vi "Auto Controller.vi"(8 "Start Position":T2, 9 "End Position":T1, 10 "Cluster":cluster{"Start Time (ms)":u32, "Iterations":i32}, 11 "RobotDriveDevRef":T3) -> (1 "Finished?":bool, 2 "Right":dbl, 3 "Left":dbl)   [LabVIEW 2016]
uses:
  <vilib>/Rock Robotics/WPI/RobotDrive/WPI_RobotDriveDevRef.ctl
  <vilib>/Rock Robotics/WPI/MotorControl/WPI_MotorControlDeviceRef.ctl
  <vilib>/Rock Robotics/WPI/MotorControl/WPI_MotorControlType.ctl
  <vilib>/Rock Robotics/SystemInterfaces/DIO/FPGA_DIOPWMChannel.ctl
  <vilib>/Rock Robotics/WPI/PWM/WPI_PWMDeadband.ctl
  Shared/AutoPositions Type Def.ctl
  Shared/AutoEndPosition Type Def.ctl
  <vilib>/Rock Robotics/WPI/Camera/WPI_CameraExposure Values.ctl
  NavX/NavX Global.vi
  <vilib>/Rock Robotics/Network Tables/NT Read Number.vi
  Framework/Robot Global Data.vi
  <vilib>/Rock Robotics/Network Tables/NT Write Number.vi
panel:
  out "Straight 3":u32
  out "Turn 3":u32
  out "Drive To Center":u32
  out "Turn 2":u32
  out "Backup 1":u32
  out "Release Gear":u32
  out "Straight 2":u32
  out "Turn 1 Correction":u32
  out "Turn 1":u32
  out "Straight 1":u32
  # "Side Gear Auto"
  # "Center Auto"
  # "Shoot Auto"
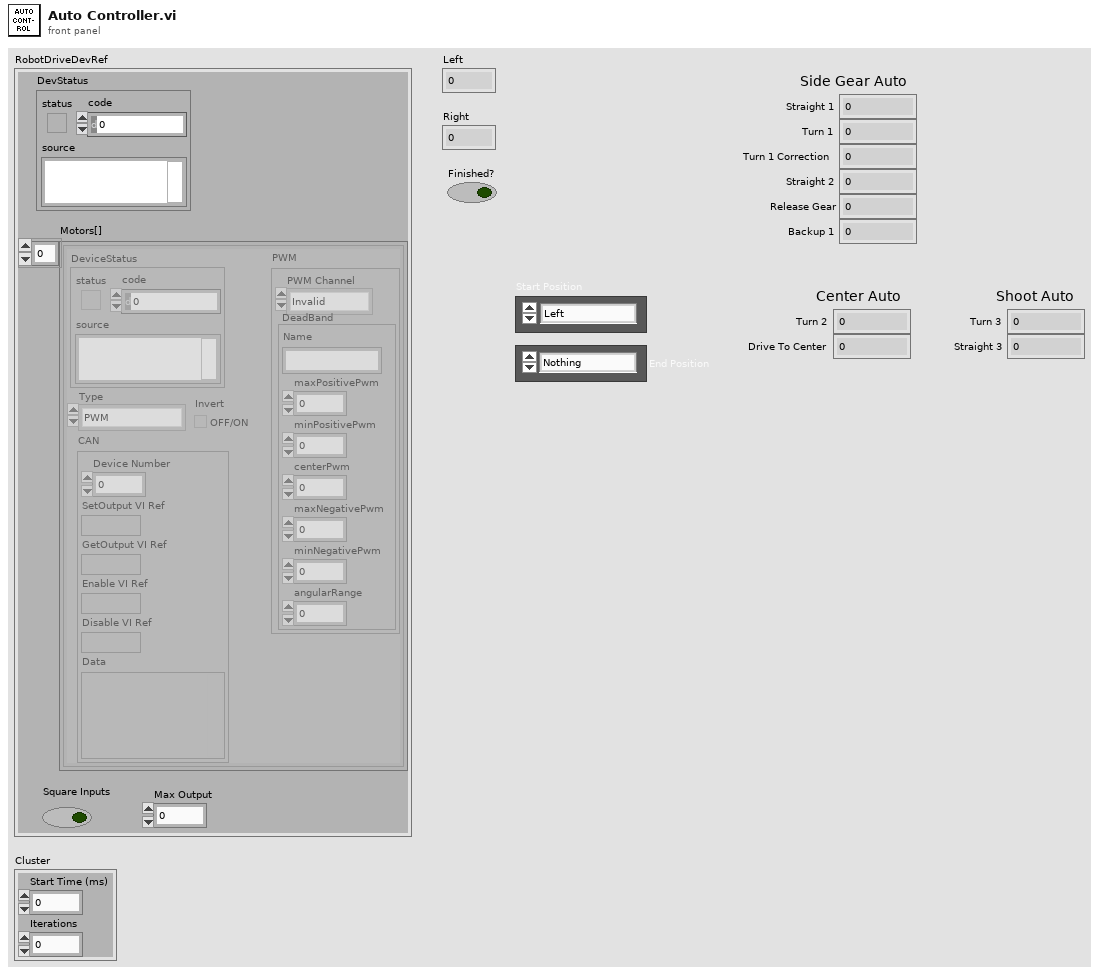
[diagram p1: front panel]
types:
  T1 = typedef "AutoEndPosition Type Def.ctl" = enum16{"Nothing", "Center", "Shoot"}
  T2 = typedef "AutoPositions Type Def.ctl" = enum16{"Left", "Middle", "Right"}
  T3 = typedef "WPI_RobotDriveDevRef.ctl" = cluster{"DevStatus":errorcluster, "Motors[]":T4[], "Square Inputs":bool, "Max Output":dbl}
  T4 = typedef "WPI_MotorControlDeviceRef.ctl" = cluster{"DeviceStatus":errorcluster, "Type":T5, "PWM":cluster{"PWM Channel":T6, "DeadBand":T7}, "CAN":cluster{"Device Number":u8, "SetOutput VI Ref":variant, "GetOutput VI Ref":variant, "Enable VI Ref":variant, "Disable VI Ref":variant, "Data":variant}, "Invert":bool}
  T5 = typedef "WPI_MotorControlType.ctl" = enum16{"PWM", "CAN"}
  T6 = typedef "FPGA_DIOPWMChannel.ctl" = enum8{"PWM 0", "PWM 1", "PWM 2", "PWM 3", "PWM 4", "PWM 5", "PWM 6", "PWM 7", "PWM 8", "PWM 9", "PWM MXP 0", "PWM MXP 1", "PWM MXP 2", "PWM MXP 3", "PWM MXP 4", "PWM MXP 5", "PWM MXP 6", "PWM MXP 7", "PWM MXP 8", "PWM MXP 9", "Invalid"}
  T7 = typedef "WPI_PWMDeadband.ctl" = cluster{"Name":string, "maxPositivePwm":i32, "minPositivePwm":i32, "centerPwm":i32, "maxNegativePwm":i32, "minNegativePwm":i32, "angularRange":u16}
  T8 = typedef "WPI_CameraExposure Values.ctl" = enum16{"Auto", "Flicker-free 50 Hz", "Flicker-free 60 Hz", "Hold current", "Custom"}
  T9 = cluster{"Yaw":dbl, "Roll":dbl, "Pitch":dbl, "Heading":dbl, "Fused Heading":dbl}
  T10 = cluster{"LinearAcceleration X":dbl, "LinearAcceleration Y":dbl, "LinearAcceleration Z":dbl}
  T11 = typedef "WPI_CameraDevRef.ctl" = cluster{"Camera Address":string, "CameraStatus":errorcluster}
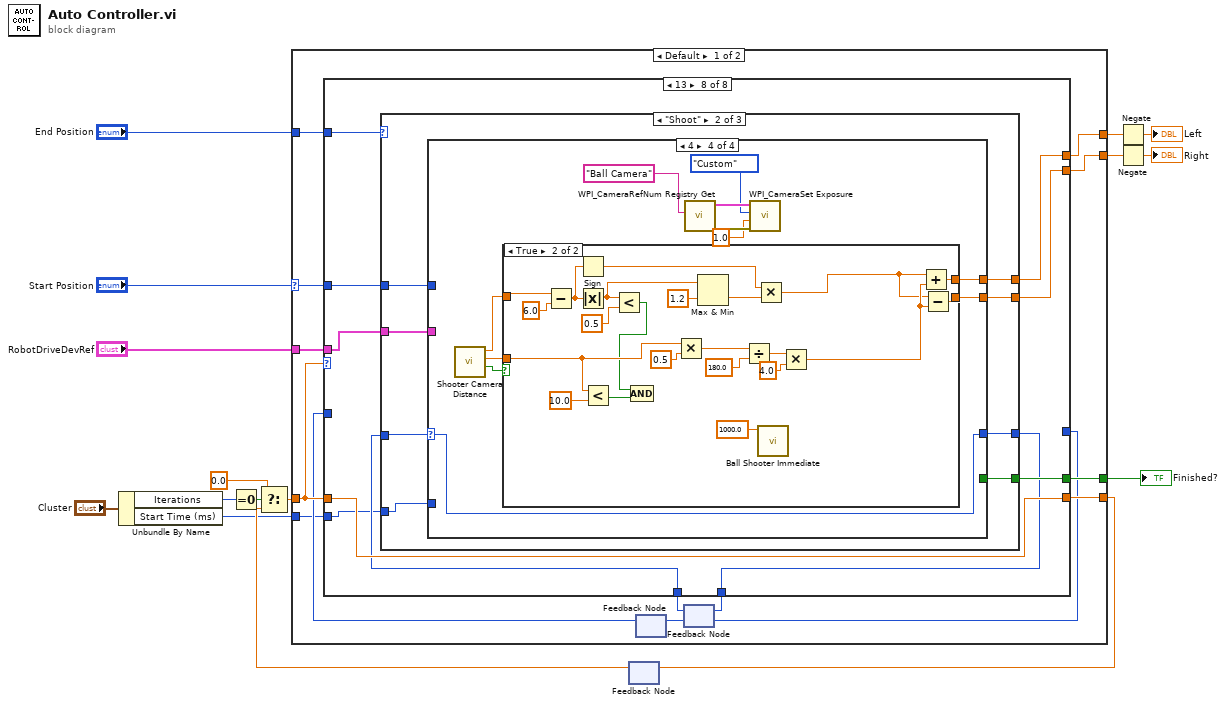
[diagram p0: block diagram]
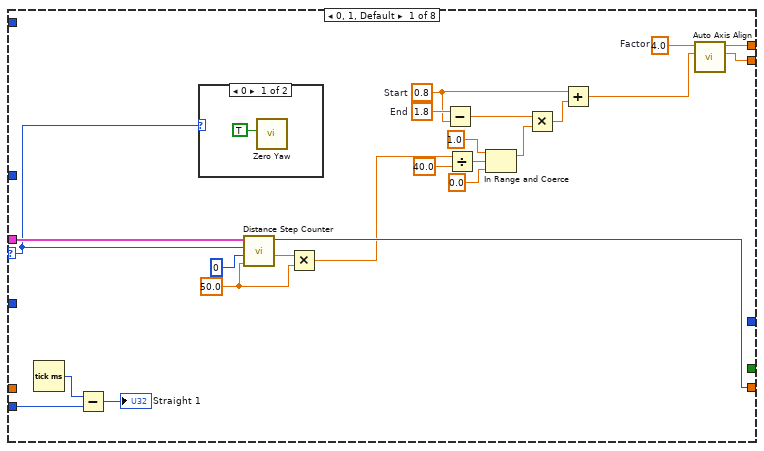
[diagram p2: hidden frame]
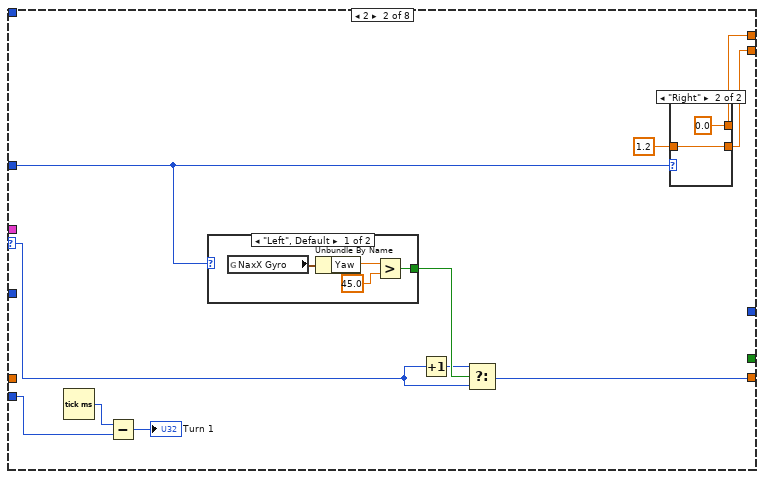
[diagram p4: hidden frame]
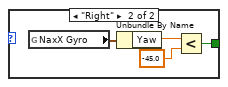
[diagram p5: hidden frame]
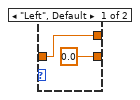
[diagram p6: hidden frame]
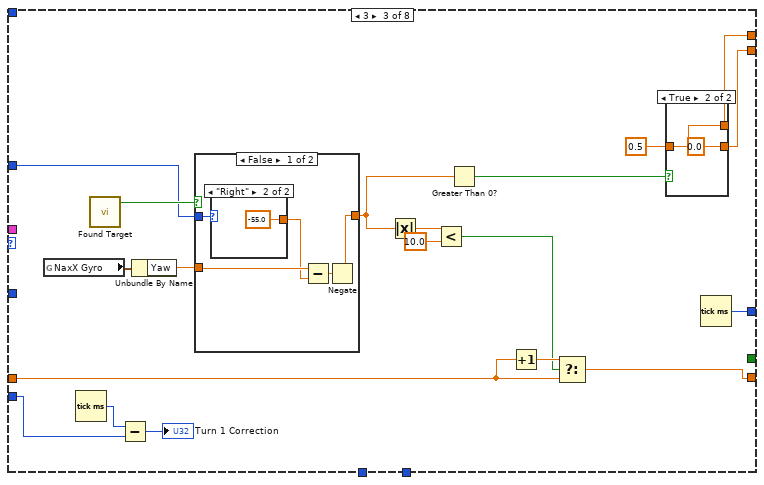
[diagram p7: hidden frame]
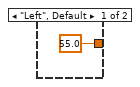
[diagram p8: hidden frame]
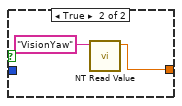
[diagram p9: hidden frame]
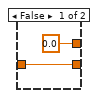
[diagram p10: hidden frame]
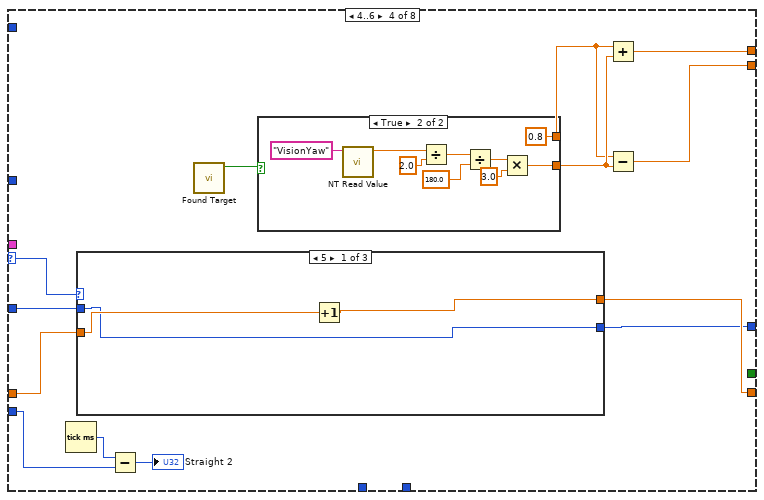
[diagram p11: hidden frame]
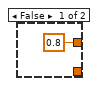
[diagram p12: hidden frame]
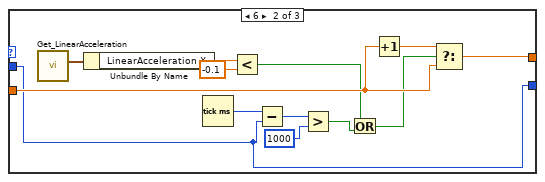
[diagram p13: hidden frame]
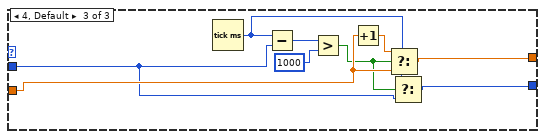
[diagram p14: hidden frame]
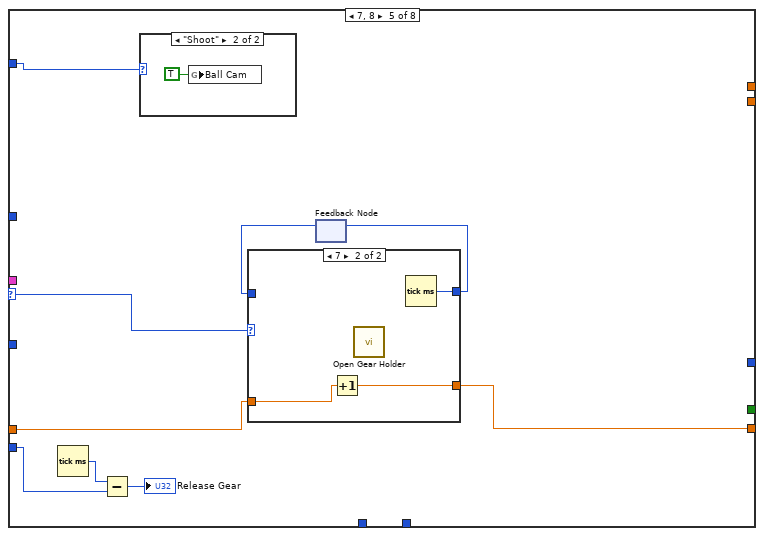
[diagram p15: hidden frame]
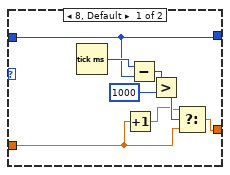
[diagram p17: hidden frame]
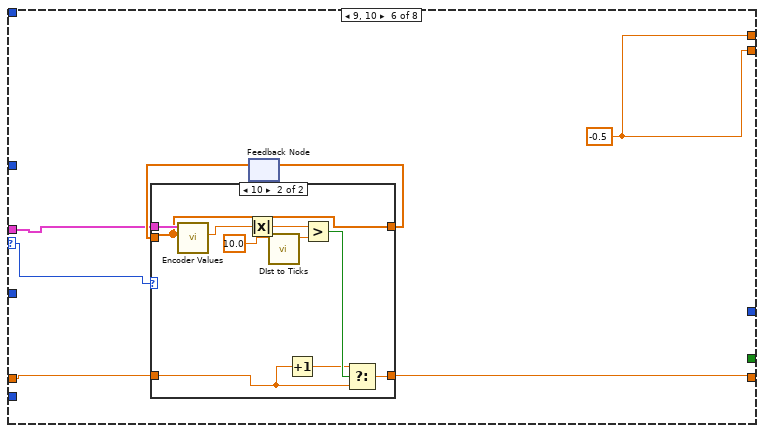
[diagram p18: hidden frame]
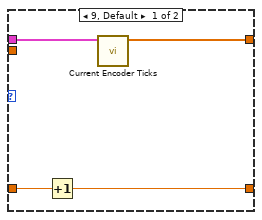
[diagram p19: hidden frame]
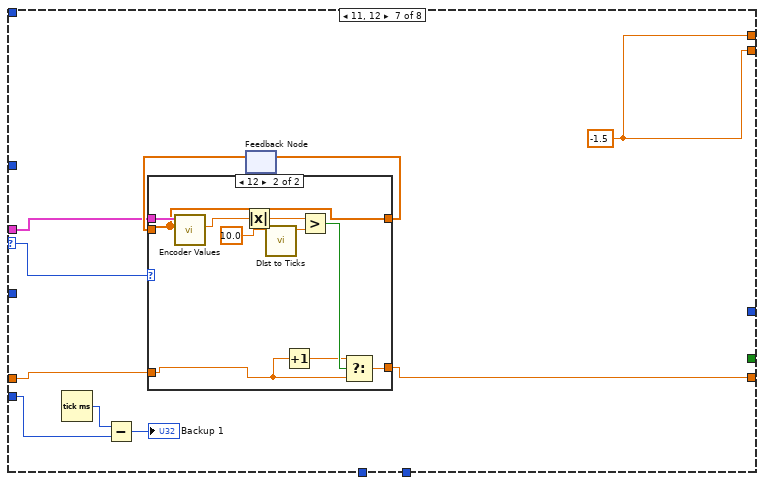
[diagram p20: hidden frame]
diagram:
  n1 = Unbundle By Name("Cluster") -> ("Iterations"=w10:i32, "Start Time (ms)"=w1:u32)
  n2 = Equal To 0?(x=w10) -> (x = 0?=w11:bool)
  n3 = feedback #1() -> (w7:dbl)  [unwired: 1 in]
  n4 = Select(t=0.0, s=w11, f=w7) -> (s? t:f=w13:dbl)
  n5 = case shown="Default" "Start Position" {
    selector: "Start Position" -> [w23 w388]
    tunnel: "RobotDriveDevRef" -> [w29 w394]
    tunnel: [w28 w393] -> w15
    tunnel: [w27 w392] -> w14
    tunnel: w13 -> [w26 w391]
    tunnel: [w25 w390] -> w8
    tunnel: [w24 w389] -> w4
    tunnel: "End Position" -> [w20 _]
    tunnel: w1 -> [w17 _]
    frame Default {
      n6 = feedback #2() -> (w21:u32)  [unwired: 1 in]
      n7 = feedback #3() -> (w19:i32)  [unwired: 1 in]
      n8 = case shown="13" w26 {
        selector: w26 -> [w47 w57 _ w118 w165 w181 w206 _]
        tunnel: w26 -> [_ _ w93 w117 w164 w182 w204 w230]
        tunnel: [w49 w62 w91 w120 _ w178 w202 w229] -> w27
        tunnel: [w48 w61 w90 w119 _ w178 w202 w228] -> w28
        tunnel: w29 -> [w52 _ _ _ _ w180 w205 w224]
        tunnel: [w51 w64 w94 w116 w163 w179 w203 w230] -> w25
        tunnel: [_ _ _ _ _ _ _ w231] -> w24
        tunnel: w23 -> [_ w63 w80 _ _ _ _ w227]
        tunnel: [_ _ w89 w114 _ _ _ _] -> w22
        tunnel: w21 -> [_ _ _ w113 _ _ _ _]
        tunnel: w20 -> [_ _ _ _ w160 _ _ w232]
        tunnel: w19 -> [_ _ _ _ _ _ _ w226]
        tunnel: [_ _ _ _ _ _ _ w225] -> w18
        tunnel: w17 -> [w31 w54 w77 w109 w157 _ w199 w223]
        frame 0, 1, Default {
          w42 = 50.0 ("Distance (in)")
          w45 = 1.8  # End
          w34 = 0.8  # Start
          w50 = 4.0  # Factor
          n9 = Tick Count (ms)() -> (millisecond timer value=w32:u32)
          n10 = Subtract(x=w32, y=w31) -> (x-y=→"Straight 1":u32)
          n11 = case shown="0" w47 {
            frame 0 {
              n12 = call <vilib>:"Zero Yaw.vi"("Zero"=TRUE) -> ()  [unwired: 11 in]
            }
            frame Default {
            }
          }
          n13 = call "Distance Step Counter.vi"("Distance (in)"=w42, "Base Step"=0, "Step"=w47, "RobotDriveDevRef"=w52) -> ("Progress"=w44:dbl, "Step out"=w51:i32)  [unwired: 5 in, 1 out]
          n14 = Multiply(x=w44, y=w42) -> (x*y=w43:dbl)
          n15 = Subtract(x=w45, y=w34) -> (x-y=w37:dbl)
          n16 = Divide(x=w43, y=40.0) -> (x/y=w40:dbl)
          n17 = In Range and Coerce(upper limit=1.0, x=w40, lower limit=0.0) -> (coerced(x)=w36:dbl)  [unwired: 1 out]
          n18 = Multiply(x=w37, y=w36) -> (x*y=w35:dbl)
          n19 = Add(x=w34, y=w35) -> (x+y=w33:dbl)
          n20 = call "Auto Axis Align.vi"("Base Speed"=w33, "Correction Factor"=w50) -> ("Right"=w48:dbl, "Left"=w49:dbl)  [unwired: 8 in]
        }
        frame 2 {
          n21 = Tick Count (ms)() -> (millisecond timer value=w56:u32)
          n22 = Subtract(x=w56, y=w54) -> (x-y=→"Turn 1":u32)
          n23 = case shown="\"Left\", Default" w63 {
            tunnel: [w65 w69] -> w59
            frame "Left", Default {
              n24 = global read "NavX Global.vi" "NaxX Gyro"() -> (w68:T9)
              n25 = Unbundle By Name(w68) -> ("Yaw"=w67:dbl)
              n26 = Greater?(x=w67, y=45.0) -> (0:w65:bool)
            }
            frame "Right" {
              n27 = global read "NavX Global.vi" "NaxX Gyro"() -> (w72:T9)
              n28 = Unbundle By Name(w72) -> ("Yaw"=w71:dbl)
              n29 = Less?(x=w71, y=-45.0) -> (x < y?=w69:bool)
            }
          }
          n30 = Increment(x=w57) -> (x+1=w58:i32)
          n31 = Select(t=w58, s=w59, f=w57) -> (s? t:f=w64:i32)
          n32 = case shown="\"Right\"" w63 {
            tunnel: [0.0 w75] -> w61
            tunnel: [w73 0.0] -> w62
            tunnel: 1.2 -> [w73 w75]
            frame "Left", Default {
            }
            frame "Right" {
            }
          }
        }
        frame 3 {
          n33 = global read "NavX Global.vi" "NaxX Gyro"() -> (w82:T9)
          n34 = Tick Count (ms)() -> (millisecond timer value=w79:u32)
          n35 = call "Found Target"() -> ("Boolean"=w83:bool)  [unwired: 11 in]
          n36 = Subtract(x=w79, y=w77) -> (x-y=→"Turn 1 Correction":u32)
          n37 = Unbundle By Name(w82) -> ("Yaw"=w81:dbl)
          n38 = case shown="False" w83 {
            tunnel: [w97 w103] -> w84
            tunnel: w81 -> [w100 _]
            tunnel: w80 -> [w98 _]
            frame False {
              n39 = case shown="\"Right\"" w98 {
                tunnel: [55.0 -55.0] -> w96
                frame "Left", Default {
                }
                frame "Right" {
                }
              }
              n40 = Subtract(x=w100, y=w96) -> (x-y=w99:dbl)
              n41 = Negate(x=w99) -> (-x=w97:dbl)
            }
            frame True {
              n42 = call-poly <vilib>:"NT Read Value.vi"("Name"="VisionYaw") -> ("Numeric"=w103:dbl)  [unwired: 9 in, 1 out]
            }
          }
          n43 = Absolute Value(x=w84) -> (abs(x)=w86:dbl)
          n44 = Less?(x=w86, y=10.0) -> (x < y?=w92:bool)
          n45 = Greater Than 0?(x=w84) -> (x > 0?=w88:bool)
          n46 = Increment(x=w93) -> (x+1=w95:dbl)
          n47 = Select(t=w95, s=w92, f=w93) -> (s? t:f=w94:dbl)
          n48 = case shown="True" w88 {
            tunnel: [w105 0.0] -> w90
            tunnel: [0.0 w107] -> w91
            tunnel: 0.5 -> [w105 w107]
            frame False {
            }
            frame True {
            }
          }
          n49 = Tick Count (ms)() -> (millisecond timer value=w89:u32)
        }
        frame 4..6 {
          n50 = Tick Count (ms)() -> (millisecond timer value=w111:u32)
          n51 = case shown="5" w118 {
            tunnel: [w132 w138 w148] -> w114
            tunnel: w113 -> [w132 w138 w149]
            tunnel: w117 -> [w133 w142 w153]
            tunnel: [w134 w144 w152] -> w116
            frame 5 {
              n52 = Increment(x=w133) -> (x+1=w134:dbl)
            }
            frame 6 {
              n53 = call <vilib>:"Get_LinearAcceleration.vi"() -> ("Linear Acceleration"=w147:T10)  [unwired: 11 in]
              n54 = Unbundle By Name(w147) -> ("LinearAcceleration X"=w146:dbl)
              n55 = Tick Count (ms)() -> (millisecond timer value=w141:u32)
              n56 = Less?(x=w146, y=-0.1) -> (x < y?=w136:bool)
              n57 = Subtract(x=w141, y=w138) -> (x-y=w140:u32)
              n58 = Greater?(x=w140, y=u32 1000) -> (0:w137:bool)
              n59 = Or(x=w136, y=w137) -> (x .or. y?=w135:bool)
              n60 = Increment(x=w142) -> (x+1=w143:dbl)
              n61 = Select(t=w143, s=w135, f=w142) -> (s? t:f=w144:dbl)
            }
            frame 4, Default {
              n62 = Tick Count (ms)() -> (millisecond timer value=w150:u32)
              n63 = Subtract(x=w150, y=w149) -> (x-y=w156:u32)
              n64 = Greater?(x=w156, y=u32 1000) -> (0:w151:bool)
              n65 = Increment(x=w153) -> (x+1=w154:dbl)
              n66 = Select(t=w154, s=w151, f=w153) -> (s? t:f=w152:dbl)
              n67 = Select(t=w150, s=w151, f=w149) -> (s? t:f=w148:u32)
            }
          }
          n68 = Subtract(x=w111, y=w109) -> (x-y=→"Straight 2":u32)
          n69 = call "Found Target"() -> ("Boolean"=w112:bool)  [unwired: 11 in]
          n70 = case shown="True" w112 {
            tunnel: [_ w127] -> w121
            tunnel: [0.8 ("x") 0.8 ("x")] -> w115
            frame False {
            }
            frame True {
              n71 = call-poly <vilib>:"NT Read Value.vi"("Name"="VisionYaw") -> ("Numeric"=w124:dbl)  [unwired: 9 in, 1 out]
              n72 = Divide(x=w124, y=2.0) -> (x/y=w128:dbl)
              n73 = Divide(x=w128, y=180.0) -> (x/y=w130:dbl)
              n74 = Multiply(x=w130, y=3.0) -> (x*y=w127:dbl)
            }
          }
          n75 = Add(x=w115, y=w121) -> (x+y=w120:dbl)
          n76 = Subtract(x=w115, y=w121) -> (x-y=w119:dbl)
        }
        frame 7, 8 {
          n77 = Tick Count (ms)() -> (millisecond timer value=w159:u32)
          n78 = Subtract(x=w159, y=w157) -> (x-y=→"Release Gear":u32)
          n79 = case shown="\"Shoot\"" w160 {
            frame "Nothing", Default {
            }
            frame "Shoot" {
              n80 = global write "Robot Global Data.vi" "Ball Cam"(TRUE ("Ball Cam")) -> ()
            }
          }
          n81 = feedback #4() -> (w161:u32)  [unwired: 1 in]
          n82 = case shown="7" w165 {
            tunnel: w164 -> [w168 w177]
            tunnel: [w170 w176] -> w163
            tunnel: [w173 w175] -> w162
            tunnel: w161 -> [w173 _]
            frame 8, Default {
              n83 = Tick Count (ms)() -> (millisecond timer value=w174:u32)
              n84 = Increment(x=w168) -> (x+1=w169:dbl)
              n85 = Subtract(x=w174, y=w173) -> (x-y=w172:u32)
              n86 = Greater?(x=w172, y=u32 1000) -> (0:w171:bool)
              n87 = Select(t=w169, s=w171, f=w168) -> (s? t:f=w170:dbl)
            }
            frame 7 {
              n88 = Increment(x=w177) -> (x+1=w176:dbl)
              n89 = call "Open Gear Holder.vi"() -> ()  [unwired: 12 in]
              n90 = Tick Count (ms)() -> (millisecond timer value=w175:u32)
            }
          }
          n91 = feedback-in #4(w162) -> ()
        }
        frame 9, 10 {
          w178 = -0.5
          n92 = feedback #5() -> (w183:dbl[])  [unwired: 1 in]
          n93 = case shown="10" w181 {
            tunnel: w180 -> [w186 w198]
            tunnel: w182 -> [w188 w193]
            tunnel: [w187 w195] -> w179
            tunnel: [w185 w191] -> w184
            tunnel: w183 -> [_ w191]
            frame 9, Default {
              n94 = Increment(x=w188) -> (x+1=w187:dbl)
              n95 = call "Current Encoder Ticks.vi"("RobotDriveDevRef"=w186) -> ("Array"=w185:dbl[])  [unwired: 10 in]
            }
            frame 10 {
              n96 = call "Encoder Values.vi"("Array"=w191, "RobotDriveDevRef"=w198) -> ("Position"=w189:dbl)  [unwired: 8 in, 1 out]
              n97 = Absolute Value(x=w189) -> (abs(x)=w190:dbl)
              n98 = call "DIst to Ticks.vi"("x"=10.0) -> ("Numeric"=w196:dbl)  [unwired: 10 in]
              n99 = Increment(x=w193) -> (x+1=w192:dbl)
              n100 = Greater?(x=w190, y=w196) -> (0:w194:bool)
              n101 = Select(t=w192, s=w194, f=w193) -> (s? t:f=w195:dbl)
            }
          }
          n102 = feedback-in #5(w184) -> ()
        }
        frame 11, 12 {
          w202 = -1.5
          n103 = Tick Count (ms)() -> (millisecond timer value=w201:u32)
          n104 = Subtract(x=w201, y=w199) -> (x-y=→"Backup 1":u32)
          n105 = feedback #6() -> (w207:dbl[])  [unwired: 1 in]
          n106 = case shown="12" w206 {
            tunnel: w205 -> [w211 w222]
            tunnel: [w212 w219] -> w203
            tunnel: [w210 w216] -> w208
            tunnel: w207 -> [_ w216]
            tunnel: w204 -> [w209 w213]
            frame 11, Default {
              n107 = Increment(x=w209) -> (x+1=w212:dbl)
              n108 = call "Current Encoder Ticks.vi"("RobotDriveDevRef"=w211) -> ("Array"=w210:dbl[])  [unwired: 10 in]
            }
            frame 12 {
              n109 = call "Encoder Values.vi"("Array"=w216, "RobotDriveDevRef"=w222) -> ("Position"=w214:dbl)  [unwired: 8 in, 1 out]
              n110 = Absolute Value(x=w214) -> (abs(x)=w215:dbl)
              n111 = call "DIst to Ticks.vi"("x"=10.0) -> ("Numeric"=w220:dbl)  [unwired: 10 in]
              n112 = Increment(x=w213) -> (x+1=w217:dbl)
              n113 = Greater?(x=w215, y=w220) -> (0:w218:bool)
              n114 = Select(t=w217, s=w218, f=w213) -> (s? t:f=w219:dbl)
            }
          }
          n115 = feedback-in #6(w208) -> ()
        }
        frame 13 {
          n116 = case shown="\"Shoot\"" w232 {
            tunnel: [TRUE w236 w342] -> w231
            tunnel: w226 -> [_ w241 w347]
            tunnel: [_ w240 w346] -> w229
            tunnel: [_ w239 w345] -> w228
            tunnel: w227 -> [_ w238 w344]
            tunnel: [_ w237 w348] -> w225
            tunnel: w224 -> [_ w235 w343]
            tunnel: w223 -> [_ w234 w341]
            frame "Nothing", Default {
            }
            frame "Shoot" {
              n117 = case shown="4" w241 {
                selector: w241 -> [_ w251 w286 w313]
                tunnel: [_ w254 w277 w316] -> w240
                tunnel: [_ w253 w276 w315] -> w239
                tunnel: w238 -> [_ w252 w272 _]
                tunnel: [1 w250 w288 w313] -> w237
                tunnel: [FALSE _ _ _] -> w236
                tunnel: w235 -> [_ _ w287 _]
                tunnel: w234 -> [_ w244 w269 _]
                frame Default {
                }
                frame 1 {
                  n118 = Tick Count (ms)() -> (millisecond timer value=w246:u32)
                  n119 = Subtract(x=w246, y=w244) -> (x-y=→"Turn 3":u32)
                  n120 = case shown="\"Right\"" w252 {
                    tunnel: [w257 w261] -> w249
                    frame "Left", Default {
                      n121 = global read "NavX Global.vi" "NaxX Gyro"() -> (w260:T9)
                      n122 = Unbundle By Name(w260) -> ("Yaw"=w259:dbl)
                      n123 = Less?(x=w259, y=-70.0) -> (x < y?=w257:bool)
                    }
                    frame "Right" {
                      n124 = global read "NavX Global.vi" "NaxX Gyro"() -> (w264:T9)
                      n125 = Unbundle By Name(w264) -> ("Yaw"=w263:dbl)
                      n126 = Greater?(x=w263, y=70.0) -> (0:w261:bool)
                    }
                  }
                  n127 = Increment(x=w251) -> (x+1=w255:i32)
                  n128 = call-poly <vilib>:"NT Write Value.vi"("Numeric"=0.0, "Name"="FoundTarget2") -> ()  [unwired: 9 in, 1 out]
                  n129 = Select(t=w255, s=w249, f=w251) -> (s? t:f=w250:i32)
                  n130 = case shown="True" w249 {
                    frame False {
                    }
                    frame True {
                      n131 = call "Auto Mode.vi"() -> ()  [unwired: 12 in]
                    }
                  }
                  n132 = case shown="\"Right\"" w252 {
                    tunnel: [0.0 w267] -> w253
                    tunnel: [w265 0.0] -> w254
                    tunnel: -1.7 -> [w265 w267]
                    frame "Left", Default {
                    }
                    frame "Right" {
                    }
                  }
                }
                frame 2, 3 {
                  w278 = 1.2
                  n133 = global read "NavX Global.vi" "NaxX Gyro"() -> (w285:T9)
                  n134 = case shown="\"Right\"" w272 {
                    tunnel: [-120.0 ("y") 120.0 ("y")] -> w274
                    frame "Left", Default {
                    }
                    frame "Right" {
                    }
                  }
                  n135 = Tick Count (ms)() -> (millisecond timer value=w271:u32)
                  n136 = Unbundle By Name(w285) -> ("Yaw"=w275:dbl)
                  n137 = Subtract(x=w271, y=w269) -> (x-y=→"Straight 3":u32)
                  n138 = Subtract(x=w275, y=w274) -> (x-y=w273:dbl)
                  n139 = feedback #7() -> (w289:dbl[])  [unwired: 1 in]
                  n140 = case shown="2, Default" w286 {
                    tunnel: w287 -> [w294 w306]
                    tunnel: w286 -> [w296 w302]
                    tunnel: [w295 w304] -> w288
                    tunnel: [w293 w300] -> w290
                    tunnel: w289 -> [_ w300]
                    frame 2, Default {
                      n141 = Increment(x=w296) -> (x+1=w295:i32)
                      n142 = call "Current Encoder Ticks.vi"("RobotDriveDevRef"=w294) -> ("Array"=w293:dbl[])  [unwired: 10 in]
                    }
                    frame 3 {
                      n143 = call "Encoder Values.vi"("Array"=w300, "RobotDriveDevRef"=w306) -> ("Position"=w298:dbl)  [unwired: 8 in, 1 out]
                      n144 = Absolute Value(x=w298) -> (abs(x)=w299:dbl)
                      n145 = call "DIst to Ticks.vi"("x"=30.0) -> ("Numeric"=w305:dbl)  [unwired: 10 in]
                      n146 = Increment(x=w302) -> (x+1=w301:i32)
                      n147 = Greater?(x=w299, y=w305) -> (0:w303:bool)
                      n148 = Select(t=w301, s=w303, f=w302) -> (s? t:f=w304:i32)
                    }
                  }
                  n149 = feedback-in #7(w290) -> ()
                  n150 = Multiply(x=w273, y=-0.5) -> (x*y=w281:dbl)
                  n151 = Divide(x=w281, y=180.0) -> (x/y=w283:dbl)
                  n152 = Multiply(x=w283, y=5.0) -> (x*y=w279:dbl)
                  n153 = Add(x=w278, y=w279) -> (x+y=w277:dbl)
                  n154 = Subtract(x=w278, y=w279) -> (x-y=w276:dbl)
                }
                frame 4 {
                  n155 = call "Shooter Camera Distance.vi"() -> ("Target Found?"=w312:bool, "Yaw"=w314:dbl, "Distance (ft)"=w317:dbl)  [unwired: 9 in]
                  n156 = case shown="True" w312 {
                    tunnel: w317 -> [_ w328]
                    tunnel: [w318 w335] -> w316
                    tunnel: [w318 w334] -> w315
                    tunnel: w314 -> [_ w333]
                    frame False {
                      w318 = 0.8
                    }
                    frame True {
                      n157 = Subtract(x=w328, y=6.0) -> (x-y=w320:dbl)
                      n158 = Sign(1:w320) -> (0:w319:dbl)
                      n159 = Absolute Value(x=w320) -> (abs(x)=w324:dbl)
                      n160 = Less?(x=w333, y=10.0) -> (x < y?=w331:bool)
                      n161 = Less?(x=w324, y=0.5) -> (x < y?=w326:bool)
                      n162 = Compound Arithmetic op=AND(w326, w331) -> ()  [unwired: 1 out]
                      n163 = Multiply(x=w333, y=0.5) -> (x*y=w337:dbl)
                      n164 = Max & Min(x=w324, y=1.2) -> (min(x,y)=w322:dbl)  [unwired: 1 out]
                      n165 = Divide(x=w337, y=180.0) -> (x/y=w339:dbl)
                      n166 = Multiply(x=w319, y=w322) -> (x*y=w321:dbl)
                      n167 = call "Ball Shooter Immediate.vi"("Duration"=1000.0) -> ()  [unwired: 10 in, 1 out]
                      n168 = Multiply(x=w339, y=4.0) -> (x*y=w330:dbl)
                      n169 = Add(x=w321, y=w330) -> (x+y=w335:dbl)
                      n170 = Subtract(x=w321, y=w330) -> (x-y=w334:dbl)
                    }
                  }
                  n171 = call <vilib>:"WPI_CameraRefNum Registry Get.vi"("refnum name"="Ball Camera") -> ("error out"=w311:errorcluster, "CameraDevRef"=w310:T11)  [unwired: 9 in]
                  n172 = call <vilib>:"WPI_CameraSet Exposure.vi"("error in (no error)"=w311, "Exposure (%)"=1.0, "Exposure"=WPI_CameraExposure_Values."Custom", "CameraDevRef"=w310) -> ()  [unwired: 8 out]
                }
              }
            }
            frame "Center" {
              n173 = case shown="2, 3" w347 {
                selector: w347 -> [_ w355 w377]
                tunnel: [_ w356 w376] -> w348
                tunnel: [_ w354 w382] -> w346
                tunnel: [_ w353 w381] -> w345
                tunnel: w344 -> [_ w352 w385]
                tunnel: w343 -> [_ _ w378]
                tunnel: [_ _ w375] -> w342
                tunnel: w341 -> [_ w349 w371]
                frame Default {
                }
                frame 0, 1 {
                  n174 = Tick Count (ms)() -> (millisecond timer value=w351:u32)
                  n175 = Subtract(x=w351, y=w349) -> (x-y=→"Turn 2":u32)
                  n176 = case shown="1" w355 {
                    selector: w355 -> [w361 w363]
                    tunnel: [w362 w370] -> w356
                    frame 0, Default {
                      n177 = call "Close Gear Holder.vi"() -> ()  [unwired: 12 in]
                      n178 = Increment(x=w361) -> (x+1=w362:i32)
                    }
                    frame 1 {
                      n179 = global read "NavX Global.vi" "NaxX Gyro"() -> (w369:T9)
                      n180 = Unbundle By Name(w369) -> ("Yaw"=w367:dbl)
                      n181 = Absolute Value(x=w367) -> (abs(x)=w365:dbl)
                      n182 = Increment(x=w363) -> (x+1=w368:i32)
                      n183 = Less?(x=w365, y=30.0) -> (x < y?=w366:bool)
                      n184 = Select(t=w368, s=w366, f=w363) -> (s? t:f=w370:i32)
                    }
                  }
                  n185 = case shown="\"Left\", Default" w352 {
                    tunnel: [0.0 -1.2] -> w353
                    tunnel: [-1.2 0.0] -> w354
                    frame "Left", Default {
                    }
                    frame "Right" {
                    }
                  }
                }
                frame 2, 3 {
                  w384 = 5.0  # Factor
                  w383 = 1.8  # Base
                  n186 = Tick Count (ms)() -> (millisecond timer value=w373:u32)
                  n187 = Subtract(x=w373, y=w371) -> (x-y=→"Drive To Center":u32)
                  n188 = case shown="\"Left\"" w385 {
                    tunnel: [15 -15] -> w380
                    frame "Left" {
                    }
                    frame Default {
                    }
                  }
                  n189 = call "Distance Step Counter.vi"("Distance (in)"=200.0, "Base Step"=2, "Step"=w377, "RobotDriveDevRef"=w378) -> ("Finished?"=w375:bool, "Step out"=w376:i32)  [unwired: 5 in, 1 out]
                  n190 = call "Auto Axis Align.vi"("Yaw"=w380, "Base Speed"=w383, "Correction Factor"=w384) -> ("Right"=w381:dbl, "Left"=w382:dbl)  [unwired: 7 in]
                }
              }
            }
          }
        }
      }
      n191 = feedback-in #2(w22) -> ()
      n192 = feedback-in #3(w18) -> ()
    }
    frame "Middle" {
      n193 = case shown="1..3, Default" w391 {
        selector: w391 -> [w401 w436 w449 w503 w525 _]
        tunnel: w391 -> [w398 w435 w454 w504 w523 _]
        tunnel: [w403 _ w452 w500 w521 _] -> w392
        tunnel: [w402 _ w451 w500 w521 _] -> w393
        tunnel: w394 -> [_ _ w453 w502 w524 _]
        tunnel: [w397 w434 w450 w501 w522 _] -> w390
        tunnel: [_ _ _ _ _ TRUE] -> w389
        tunnel: w388 -> [_ _ _ _ _ _]
        frame 1..3, Default {
          w396 = 0.8 ("x")
          n194 = call "Found Target"() -> ("Boolean"=w395:bool)  [unwired: 11 in]
          n195 = case shown="False" w395 {
            tunnel: [_ w412] -> w404
            frame False {
            }
            frame True {
              n196 = call-poly <vilib>:"NT Read Value.vi"("Name"="VisionYaw") -> ("Numeric"=w405:dbl)  [unwired: 9 in, 1 out]
              n197 = Multiply(x=w405, y=0.5) -> (x*y=w408:dbl)
              n198 = Divide(x=w408, y=180.0) -> (x/y=w410:dbl)
              n199 = Multiply(x=w410, y=4.0) -> (x*y=w412:dbl)
            }
          }
          n200 = feedback #8() -> (w399:u32)  [unwired: 1 in]
          n201 = case shown="3" w401 {
            tunnel: [w413 w421 w431] -> w400
            tunnel: w399 -> [w413 w421 _]
            tunnel: w398 -> [w415 w422 w430]
            tunnel: [w416 w423 w429] -> w397
            frame 2 {
              n202 = Tick Count (ms)() -> (millisecond timer value=w420:u32)
              n203 = Subtract(x=w420, y=w413) -> (x-y=w419:u32)
              n204 = Greater?(x=w419, y=u32 500) -> (0:w417:bool)
              n205 = Increment(x=w415) -> (x+1=w414:dbl)
              n206 = Select(t=w414, s=w417, f=w415) -> (s? t:f=w416:dbl)
            }
            frame 3 {
              n207 = Tick Count (ms)() -> (millisecond timer value=w428:u32)
              n208 = Subtract(x=w428, y=w421) -> (x-y=w427:u32)
              n209 = Greater?(x=w427, y=u32 5000) -> (0:w425:bool)
              n210 = Increment(x=w422) -> (x+1=w424:dbl)
              n211 = Select(t=w424, s=w425, f=w422) -> (s? t:f=w423:dbl)
            }
            frame 1, Default {
              n212 = Increment(x=w430) -> (x+1=w429:dbl)
              n213 = Tick Count (ms)() -> (millisecond timer value=w431:u32)
            }
          }
          n214 = feedback-in #8(w400) -> ()
          n215 = Add(x=w396, y=w404) -> (x+y=w403:dbl)
          n216 = Subtract(x=w396, y=w404) -> (x-y=w402:dbl)
        }
        frame 4, 5 {
          n217 = feedback #9() -> (w432:u32)  [unwired: 1 in]
          n218 = case shown="4" w436 {
            tunnel: w435 -> [w438 w447]
            tunnel: [w440 w446] -> w434
            tunnel: [w443 w445] -> w433
            tunnel: w432 -> [w443 _]
            frame 5, Default {
              n219 = Tick Count (ms)() -> (millisecond timer value=w444:u32)
              n220 = Increment(x=w438) -> (x+1=w439:dbl)
              n221 = Subtract(x=w444, y=w443) -> (x-y=w442:u32)
              n222 = Greater?(x=w442, y=u32 1000) -> (0:w441:bool)
              n223 = Select(t=w439, s=w441, f=w438) -> (s? t:f=w440:dbl)
            }
            frame 4 {
              n224 = Increment(x=w447) -> (x+1=w446:dbl)
              n225 = call "Open Gear Holder.vi"() -> ()  [unwired: 12 in]
              n226 = Tick Count (ms)() -> (millisecond timer value=w445:u32)
            }
          }
          n227 = feedback-in #9(w433) -> ()
        }
        frame 6, 7 {
          n228 = case shown="True" FALSE {
            tunnel: w454 -> [w456 w470]
            tunnel: w453 -> [_ w469]
            tunnel: [_ w465] -> w452
            tunnel: [_ w464] -> w451
            tunnel: [w455 w458] -> w450
            tunnel: w449 -> [_ w457]
            frame False {
              n229 = Increment(x=w456) -> (x+1=w455:dbl)
            }
            frame True {
              n230 = feedback #10() -> (w471:dbl[])  [unwired: 1 in]
              n231 = feedback #11() -> (w468:i32)  [unwired: 1 in]
              n232 = case shown="7" w457 {
                tunnel: w469 -> [w475 w479]
                tunnel: w470 -> [w477 w478]
                tunnel: [w476 w478] -> w459
                tunnel: [w474 w480] -> w472
                tunnel: w471 -> [_ w481]
                tunnel: w468 -> [_ w482]
                tunnel: [0 w483] -> w462
                frame 6, Default {
                  n233 = Increment(x=w477) -> (x+1=w476:dbl)
                  n234 = call "Current Encoder Ticks.vi"("RobotDriveDevRef"=w475) -> ("Array"=w474:dbl[])  [unwired: 10 in]
                }
                frame 7 {
                  n235 = call "Encoder Values.vi"("Array"=w481, "RobotDriveDevRef"=w479) -> ("Position"=w485:dbl)  [unwired: 8 in, 1 out]
                  n236 = Absolute Value(x=w485) -> (abs(x)=w486:dbl)
                  n237 = call "DIst to Ticks.vi"("x"=0.0) -> ("Numeric"=w487:dbl)  [unwired: 10 in]
                  n238 = Greater?(x=w486, y=w487) -> (0:w484:bool)
                  n239 = case shown="True" w484 {
                    tunnel: [w490 w494] -> w483
                    tunnel: w482 -> [w490 w493]
                    tunnel: w481 -> [w489 _]
                    tunnel: [w489 w491] -> w480
                    tunnel: w479 -> [_ w492]
                    frame False {
                    }
                    frame True {
                      n240 = call "Current Encoder Ticks.vi"("RobotDriveDevRef"=w492) -> ("Array"=w491:dbl[])  [unwired: 10 in]
                      n241 = Increment(x=w493) -> (x+1=w494:i32)
                    }
                  }
                }
              }
              n242 = feedback-in #10(w472) -> ()
              n243 = feedback-in #11(w462) -> ()
              n244 = Quotient & Remainder(x=w462, y=2) -> (x-y*floor(x/y)=w466:i32)  [unwired: 1 out]
              n245 = Greater?(x=w462, y=4) -> (0:w460:bool)
              n246 = Increment(x=w459) -> (x+1=w463:dbl)
              n247 = case shown="7" w457 {
                tunnel: w466 -> [_ w497]
                tunnel: [_ w496] -> w465
                tunnel: [_ w495] -> w464
                frame Default {
                }
                frame 7 {
                  n248 = case shown="0, Default" w497 {
                    tunnel: [w498 w499] -> w496
                    tunnel: [w498 w499] -> w495
                    frame 0, Default {
                      w498 = -0.8 ("y")
                    }
                    frame 1 {
                      w499 = 0.8 ("y")
                    }
                  }
                }
              }
              n249 = Select(t=w463, s=w460, f=w459) -> (s? t:f=w458:dbl)
            }
          }
        }
        frame 8, 9 {
          w500 = -0.5
          n250 = feedback #12() -> (w505:dbl[])  [unwired: 1 in]
          n251 = case shown="9" w503 {
            tunnel: w502 -> [w508 w520]
            tunnel: w504 -> [w510 w515]
            tunnel: [w509 w517] -> w501
            tunnel: [w507 w513] -> w506
            tunnel: w505 -> [_ w513]
            frame 8, Default {
              n252 = Increment(x=w510) -> (x+1=w509:dbl)
              n253 = call "Current Encoder Ticks.vi"("RobotDriveDevRef"=w508) -> ("Array"=w507:dbl[])  [unwired: 10 in]
            }
            frame 9 {
              n254 = call "Encoder Values.vi"("Array"=w513, "RobotDriveDevRef"=w520) -> ("Position"=w511:dbl)  [unwired: 8 in, 1 out]
              n255 = Absolute Value(x=w511) -> (abs(x)=w512:dbl)
              n256 = call "DIst to Ticks.vi"("x"=10.0) -> ("Numeric"=w518:dbl)  [unwired: 10 in]
              n257 = Increment(x=w515) -> (x+1=w514:dbl)
              n258 = Greater?(x=w512, y=w518) -> (0:w516:bool)
              n259 = Select(t=w514, s=w516, f=w515) -> (s? t:f=w517:dbl)
            }
          }
          n260 = feedback-in #12(w506) -> ()
        }
        frame 10, 11 {
          w521 = -1.0
          n261 = feedback #13() -> (w526:dbl[])  [unwired: 1 in]
          n262 = case shown="11" w525 {
            tunnel: w524 -> [w530 w541]
            tunnel: [w531 w538] -> w522
            tunnel: [w529 w535] -> w527
            tunnel: w526 -> [_ w535]
            tunnel: w523 -> [w528 w532]
            frame 10, Default {
              n263 = Increment(x=w528) -> (x+1=w531:dbl)
              n264 = call "Current Encoder Ticks.vi"("RobotDriveDevRef"=w530) -> ("Array"=w529:dbl[])  [unwired: 10 in]
            }
            frame 11 {
              n265 = call "Encoder Values.vi"("Array"=w535, "RobotDriveDevRef"=w541) -> ("Position"=w533:dbl)  [unwired: 8 in, 1 out]
              n266 = Absolute Value(x=w533) -> (abs(x)=w534:dbl)
              n267 = call "DIst to Ticks.vi"("x"=40.0) -> ("Numeric"=w539:dbl)  [unwired: 10 in]
              n268 = Increment(x=w532) -> (x+1=w536:dbl)
              n269 = Greater?(x=w534, y=w539) -> (0:w537:bool)
              n270 = Select(t=w536, s=w537, f=w532) -> (s? t:f=w538:dbl)
            }
          }
          n271 = feedback-in #13(w527) -> ()
        }
        frame 12 {
        }
      }
    }
  }
  "Finished?" <- w4
  n272 = feedback-in #1(w8) -> ()
  n273 = Negate(x=w14) -> (-x=→"Left":dbl)
  n274 = Negate(x=w15) -> (-x=→"Right":dbl)
